vi "comm get handles.vi"(8 "error in (no error)":errorcluster) -> (0 "error out":errorcluster, 3 "handles":u32[](array[numeric]))   [LabVIEW 2017, in "lvserial.lvlib"]
doc: "This function returns the handles of all actually opened serial ports."
uses:
  lvserial.lvlib
  lvserial.dll
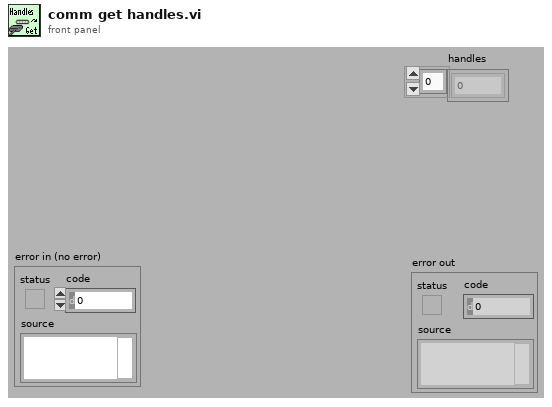
[diagram p1: front panel]
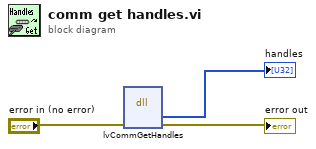
[diagram p0: block diagram]
diagram:
  n1 = dll-call lib="lvserial.dll" fn="lvCommGetHandles"("error in (no error)"="error in (no error)") -> ("phaulHandles"=→"handles":u32[], "error in (no error)"=→"error out":errorcluster)  [unwired: 3 in, 4 out]
